vi "Previous_Folder.vi"(11 "Path in":path) -> (3 "Path out":path)   [LabVIEW 2012]
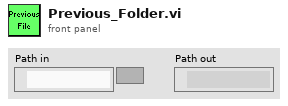
[diagram p1: front panel]
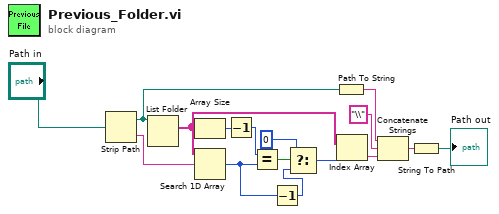
[diagram p0: block diagram]
diagram:
  n1 = Strip Path(path="Path in") -> (stripped path=w6:path, name=w1:string)
  n2 = List Folder(path=w6) -> (filenames=w9:string[])  [unwired: 3 in, 3 out]
  n3 = Array Size(array=w9) -> (size(s)=w2:i32)
  n4 = Search 1D Array(1D array=w9, element=w1) -> (index of element=w14:i32)  [unwired: 1 in]
  n5 = Decrement(x=w2) -> (x-1=w3:i32)
  n6 = Equal?(x=w3, y=w14) -> (x = y?=w12:bool)
  n7 = Decrement(x=w14) -> (x-1=w13:i32)
  n8 = Select(t=0, s=w12, f=w13) -> (s? t:f=w16:i32)
  n9 = Path To String(path=w6) -> (string=w5:string)
  n10 = Index Array(array=w9, index=w16) -> (element=w4:string)
  n11 = Concatenate Strings(w5, "\\", w4) -> (w8:string)
  n12 = String To Path(string=w8) -> (path=→"Path out":path)
